vi "USB_DAQ__EEPROM_Test_Array_Read_24C32.vi"() -> ()   [LabVIEW 2022 SP3]
panel:
  in  "stop":bool
  out "Rx.Array.Out":u8[](array[numeric])=[255, 255, 255, 255, 255, 255, 255, 255] format="%02x"
  in  "Page.Address.0":u8 format="%02x"
  out "Page.ACK.0":bool
  out "Addr.ACK.2":bool
  in  "Page.Address.1":u8 format="%02x"
  out "Page.ACK.1":bool
  out "Addr.ACK.1":bool
  in  "24C32.Address":u8=87 format="%02x"
  in  "Read":bool
  # "EEPROM 24C32 ARRAY READ"
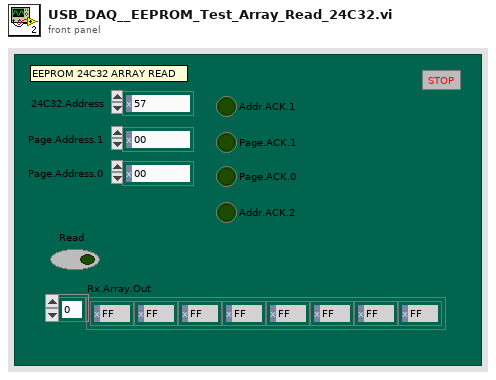
[diagram p1: front panel]
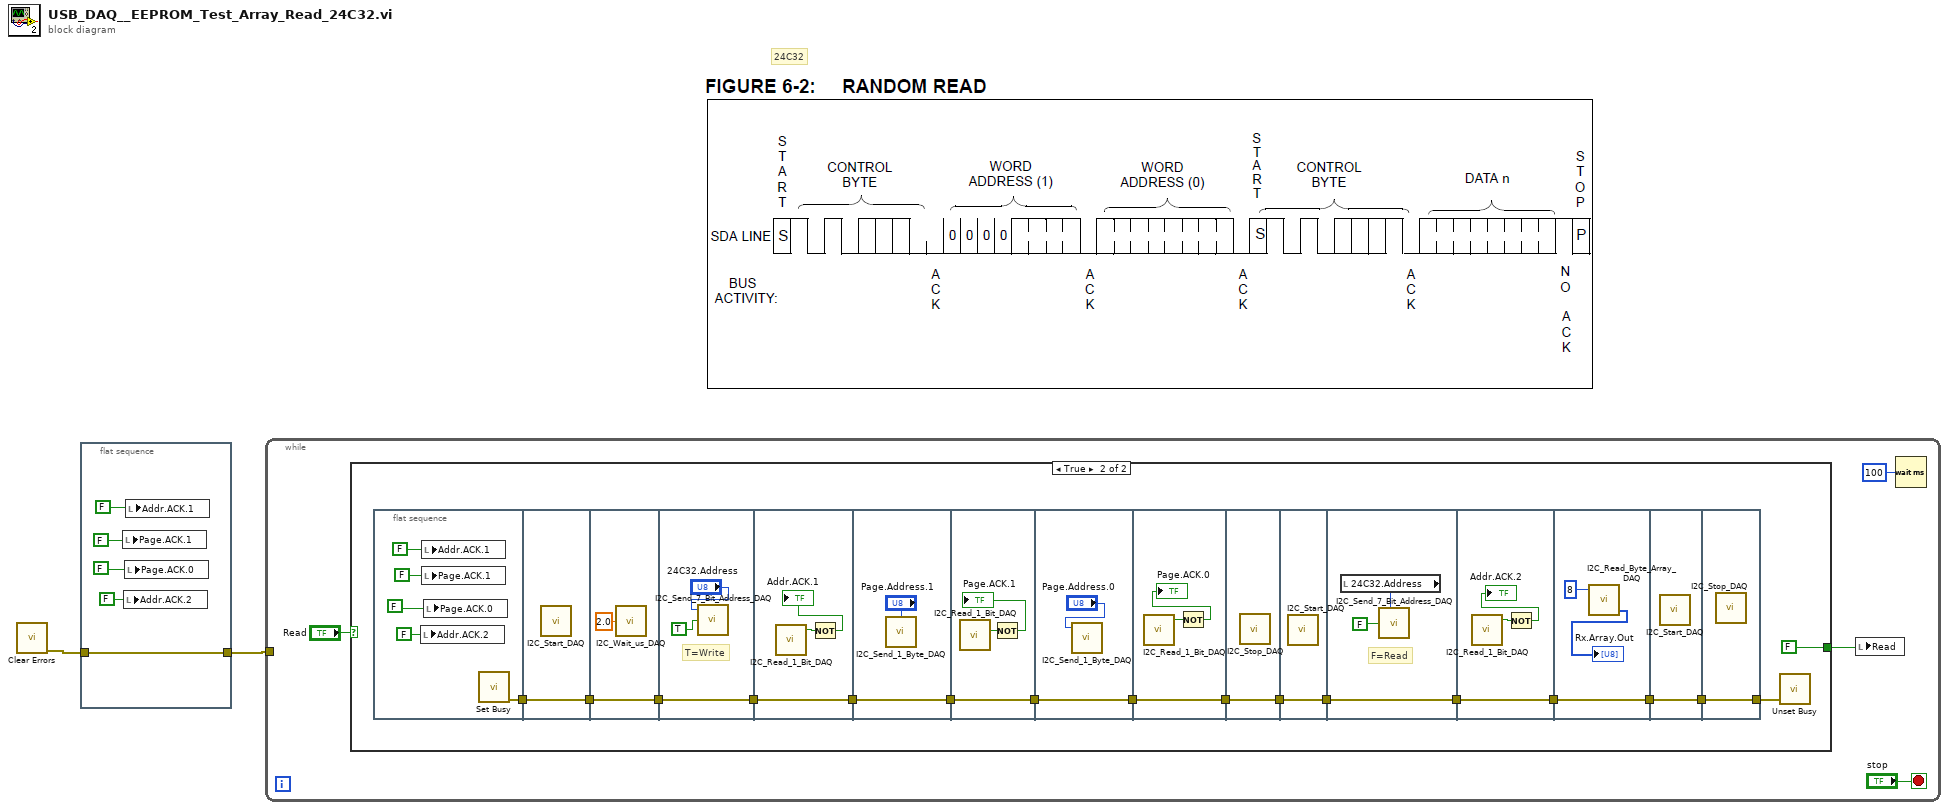
[diagram p0: block diagram]
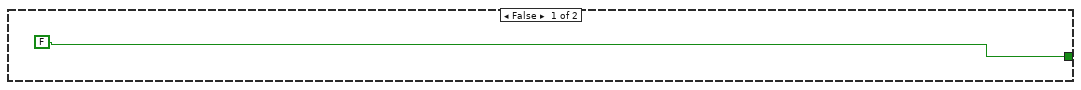
[diagram p2: hidden frame]
diagram:
  # "24C32"
  n1 = call <vilib>:"Clear Errors.vi"() -> ("error out"=w1:errorcluster)  [unwired: 6 in, 1 out]
  n2 = flat-sequence {
    tunnel: w1 -> [w7]
    tunnel: [w7] -> w2
    frame #0 {
      n3 = local write "Page.ACK.1"(FALSE ("TX.ACK")) -> ()
      n4 = local write "Addr.ACK.2"(FALSE ("Addr.ACK.2")) -> ()
      n5 = local write "Page.ACK.0"(FALSE ("Page.ACK.0")) -> ()
      n6 = local write "Addr.ACK.1"(FALSE ("ACK_OK")) -> ()
    }
  }
  n7 = while {
    tunnel: w2 -> [_]
    stop <- "stop" stop-if-true
    n8 = case shown="True" "Read" {
      tunnel: [FALSE ("Test") FALSE ("Test")] -> w9
      frame False {
      }
      frame True {
        n9 = flat-sequence {
          tunnel: [w30] -> w14
          tunnel: [w35] -> w15
          tunnel: w14 -> [w35]
          tunnel: [w36] -> w16
          tunnel: w15 -> [w36]
          tunnel: [w38] -> w17
          tunnel: w16 -> [w38]
          tunnel: [w41] -> w18
          tunnel: w17 -> [w41]
          tunnel: [w44] -> w19
          tunnel: w18 -> [w44]
          tunnel: [w46] -> w20
          tunnel: w19 -> [w46]
          tunnel: [w49] -> w21
          tunnel: w20 -> [w49]
          tunnel: [w51] -> w22
          tunnel: w21 -> [w51]
          tunnel: [w54] -> w23
          tunnel: w22 -> [w54]
          tunnel: [w55] -> w24
          tunnel: w23 -> [w55]
          tunnel: [w56] -> w25
          tunnel: w24 -> [w56]
          tunnel: [w59] -> w26
          tunnel: w25 -> [w59]
          tunnel: [w62] -> w27
          tunnel: w26 -> [w62]
          tunnel: [w65] -> w28
          tunnel: w27 -> [w65]
          tunnel: w28 -> [w66]
          tunnel: [w66] -> w13
          frame #0 {
            n10 = local write "Addr.ACK.2"(FALSE ("Addr.ACK.2")) -> ()
            n11 = local write "Addr.ACK.1"(FALSE ("ACK_OK")) -> ()
            n12 = local write "Page.ACK.1"(FALSE ("TX.ACK")) -> ()
            n13 = local write "Page.ACK.0"(FALSE ("Page.ACK.0")) -> ()
            n14 = call <vilib>:"Set Busy.vi"() -> ("error out"=w30:errorcluster)  [unwired: 10 in, 1 out]
          }
          frame #1 {
            n15 = call "I2C_Start_DAQ.vi"() -> ()  [unwired: 6 in]
          }
          frame #2 {
            n16 = call "I2C_Wait_us_DAQ.vi"("Factor"=2.0) -> ()  [unwired: 5 in]
          }
          frame #3 {
            # "T=Write"
            n17 = call "I2C_Send_7_Bit_Address_DAQ.vi"("Write or Read?"=TRUE, "Receiver_7_Bit_Address"="24C32.Address") -> ()  [unwired: 1 in]
          }
          frame #4 {
            n18 = call "I2C_Read_1_Bit_DAQ.vi"() -> ("RX_Bit_Out"=w43:bool)  [unwired: 2 in]
            n19 = Not(x=w43) -> (.not. x?=→"Addr.ACK.1":bool)
          }
          frame #5 {
            n20 = call "I2C_Send_1_Byte_DAQ.vi"("Byte_To_Send"="Page.Address.1") -> ()  [unwired: 2 in]
          }
          frame #6 {
            n21 = call "I2C_Read_1_Bit_DAQ.vi"() -> ("RX_Bit_Out"=w48:bool)  [unwired: 2 in]
            n22 = Not(x=w48) -> (.not. x?=→"Page.ACK.1":bool)
          }
          frame #7 {
            n23 = call "I2C_Send_1_Byte_DAQ.vi"("Byte_To_Send"="Page.Address.0") -> ()  [unwired: 2 in]
          }
          frame #8 {
            n24 = call "I2C_Read_1_Bit_DAQ.vi"() -> ("RX_Bit_Out"=w53:bool)  [unwired: 2 in]
            n25 = Not(x=w53) -> (.not. x?=→"Page.ACK.0":bool)
          }
          frame #9 {
            n26 = call "I2C_Stop_DAQ.vi"() -> ()  [unwired: 6 in]
          }
          frame #10 {
            n27 = call "I2C_Start_DAQ.vi"() -> ()  [unwired: 6 in]
          }
          frame #11 {
            # "F=Read"
            n28 = local read "24C32.Address"() -> (w57:u8)
            n29 = call "I2C_Send_7_Bit_Address_DAQ.vi"("Write or Read?"=FALSE, "Receiver_7_Bit_Address"=w57) -> ()  [unwired: 1 in]
          }
          frame #12 {
            n30 = call "I2C_Read_1_Bit_DAQ.vi"() -> ("RX_Bit_Out"=w61:bool)  [unwired: 2 in]
            n31 = Not(x=w61) -> (.not. x?=→"Addr.ACK.2":bool)
          }
          frame #13 {
            n32 = call "I2C_Read_Byte_Array_DAQ.vi"("Rx.Byte.Count.In"=8) -> ("Rx.Array.Out"=→"Rx.Array.Out":u8[])  [unwired: 1 in]
          }
          frame #14 {
            n33 = call "I2C_Start_DAQ.vi"() -> ()  [unwired: 6 in]
          }
          frame #15 {
            n34 = call "I2C_Stop_DAQ.vi"() -> ()  [unwired: 6 in]
          }
        }
        n35 = call <vilib>:"Unset Busy.vi"("error in (no error)"=w13) -> ()  [unwired: 10 in, 1 out]
      }
    }
    n36 = local write "Read"(w9) -> ()
    n37 = Wait (ms)(milliseconds to wait=u32 100) -> ()  [unwired: 1 out]
  }
